vi "RSZVB Set Trace Format.vi"(8 "error in (no error)":errorcluster {"code" format="%.0x"}, 9 "Format (0: dB Mag)":i32(ring) items=["dB Mag", "Phase", "Smith", "Polar", "Delay", "SWR", "Lin Mag", "Real", "Imag", "Inverted Smith", "Unwrapped Phase"], 10 "Channel (Trace) (1)":i32=1, 11 "VISA session":refnum<visa-resource-name>) -> (0 "error out":errorcluster {"code" format="%.0x"}, 3 "dup VISA session":refnum<visa-resource-name>)   [LabVIEW 2015]
doc: "This VI defines how the measured result at any sweep point is post-processed and presented in the graphical display.\n\nNote(s):\n\nThe analyzer allows arbitrary combinations of display formats and measured quantities. Nevertheless, it is advisable to check which display formats are generally appropriate for an analysis of a particular measured quantity.\n\nRemote-control command(s):\nCALCulate<Ch/Tr>:FORMat MLINear | MLOGarithmic | PHASe | UPHase | POLar | SMITh | ISMith | GDELay | REAL | IMAGinary | SWR | COMPlex | MAGNitude"
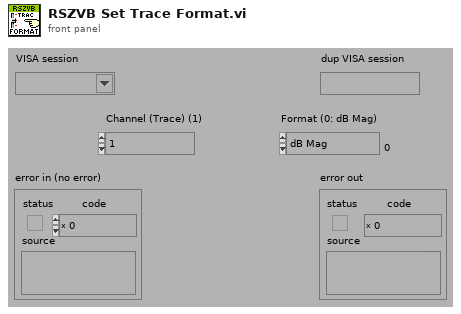
[diagram p1: front panel]
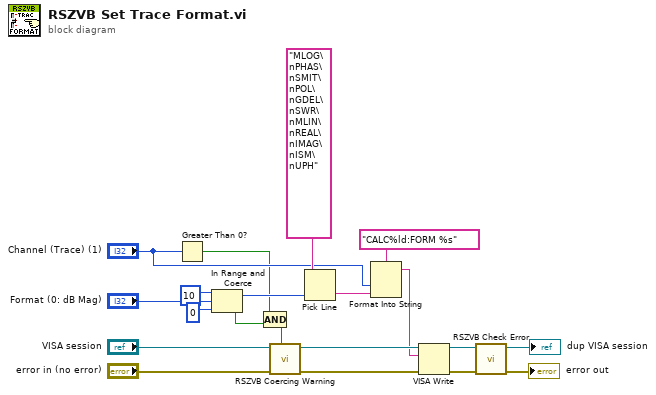
[diagram p0: block diagram]
diagram:
  n1 = Greater Than 0?(x="Channel (Trace) (1)") -> (x > 0?=w3:bool)
  n2 = In Range and Coerce(upper limit=10, x="Format (0: dB Mag)", lower limit=0) -> (coerced(x)=w17:i32, In Range?=w4:bool)
  n3 = Compound Arithmetic op=AND(w3, w4) -> (w2:bool)
  n4 = call "RSZVB Coercing Warning.vi"("In Range?"=w2, "error in (no error)"="error in (no error)", "VISA session"="VISA session") -> ("error out"=w14:errorcluster, "dup VISA session"=w15:refnum<visa-resource-name>)  [unwired: 7 in]
  n5 = Pick Line(multi-line string="MLOG\nPHAS\nSMIT\nPOL\nGDEL\nSWR\nMLIN\nREAL\nIMAG\nISM\nUPH", line index=w17) -> (output string=w6:string)  [unwired: 1 in]
  n6 = Format Into String(format string="CALC%ld:FORM %s", "Channel (Trace) (1)", w6) -> (resulting string=w1:string)  [unwired: 2 in, 1 out]
  n7 = VISA Write(VISA resource name=w15, write buffer=w1, error in (no error)=w14) -> (VISA resource name out=w12:refnum<visa-resource-name>, error out=w13:errorcluster)  [unwired: 1 out]
  n8 = call "RSZVB Check Error.vi"("error in (no error)"=w13, "VISA session"=w12) -> ("error out"=→"error out":errorcluster, "dup VISA session"=→"dup VISA session":refnum<visa-resource-name>)  [unwired: 8 in]
